vi "get_set_opv.vi"(8 "error in (no error)":errorcluster, 10 "Channel":string="1", 11 "VISA Refnum in":refnum<visa-resource-name>) -> (0 "error out":errorcluster, 2 "Set OPV (A)":string, 3 "VISA Refnum out":refnum<visa-resource-name>)   [LabVIEW 2018]
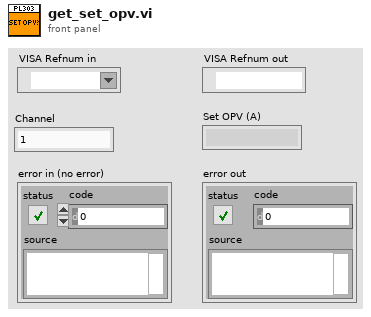
[diagram p1: front panel]
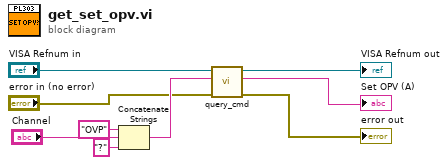
[diagram p0: block diagram]
diagram:
  n1 = Concatenate Strings("OVP" ("string"), "Channel", "?" ("string")) -> (w3:string)
  n2 = call "query_cmd.vi"("error in (no error)"="error in (no error)", "write buffer"=w3, "VISA Refnum in"="VISA Refnum in") -> ("error out"=→"error out":errorcluster, "String"=→"Set OPV (A)":string, "VISA Refnum out"=→"VISA Refnum out":refnum<visa-resource-name>)  [unwired: 6 in]
